vi "LCB Get Extended Last Error String.vi"(8 "error in (no error)":errorcluster caption="Fehler (Eingang, kein Fehler)") -> (0 "error out":errorcluster caption="Fehler (Ausgang)", 3 "Error Message":string)   [LabVIEW 2023, in "labbCAN_Bus_API.lvlib"]
doc: "LCB_Func long __stdcall LCB_GetDevErrMsg(dev_hdl hDev,\n unsigned long DevErr,\n char *pMsgBuf,\n int MsgBufSize);"
uses:
  labbCAN_Bus_API.lvlib
  labbCAN_Bus_API.dll
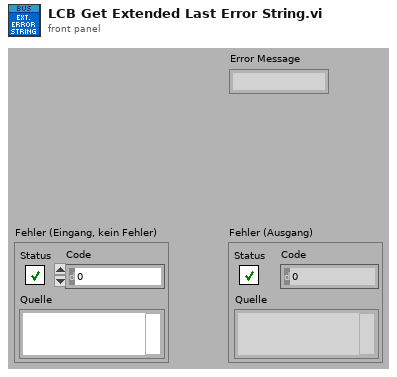
[diagram p1: front panel]
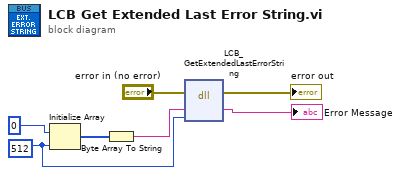
[diagram p0: block diagram]
diagram:
  w2 = 512 ("Dimension")
  n1 = Initialize Array(u8 0 ("Element"), w2) -> (w7:u8[])
  n2 = Byte Array To String(unsigned byte array=w7) -> (string=w6:string)
  n3 = dll-call lib="C:/GIT/DensityGradientProject/CETONI_SDK/labbCAN_Bus_API.*" fn="LCB_GetExtendedLastErrorString"(error in="error in (no error)", "pStringBuf"=w6, "StringBufSize"=w2) -> (error out=→"error out":errorcluster, "pStringBuf"=→"Error Message":string)  [unwired: 4 in, 1 out]
